vi "Configure.vi"(7 "Task Ident":string, 8 "error in":errorcluster, 9 "Task-Point Idents":string[](array[string]), 10 "MSS":refnum<class "Measure and Stimulus Subsystems.lvclass">, 11 "ITask Actor in":refnum<class "Task Actor.lvclass">) -> (0 "error out":errorcluster, 3 "ITask Actor out":refnum<class "Task Actor.lvclass">)   [LabVIEW 2023, in "Task Actor.lvlib" / "Task Actor.lvclass"]
uses:
  Task Actor.lvclass
  Measure and Stimulus Subsystems/Measure and Stimulus Subsystems.lvclass
  Task Actor.lvclass/Task Actor.ctl
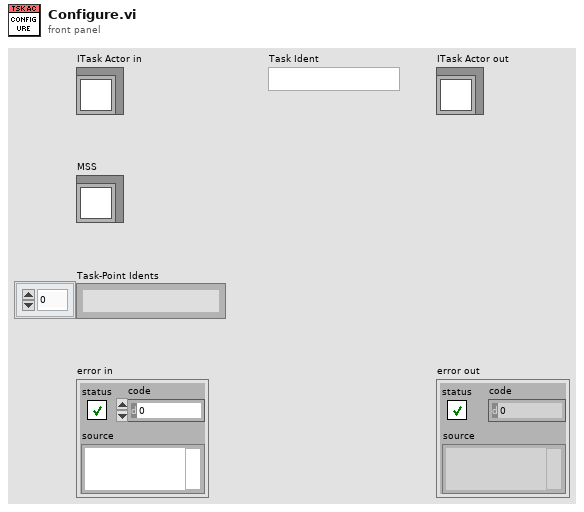
[diagram p1: front panel]
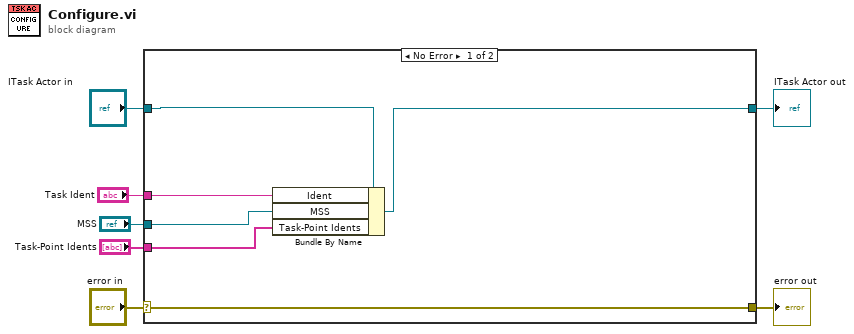
[diagram p0: block diagram]
diagram:
  n1 = case shown="No Error" "error in" {
    selector: "error in" -> [w13 w15]
    tunnel: [w13 w15] -> w6
    tunnel: [w11 w14] -> w4
    tunnel: "ITask Actor in" -> [w12 w14]
    tunnel: "Task Ident" -> [w10 _]
    tunnel: "MSS" -> [w9 _]
    tunnel: "Task-Point Idents" -> [w8 _]
    frame No Error {
      n2 = Bundle By Name(cluster=w12, "Ident"=w10, "MSS"=w9, "Task-Point Idents"=w8) -> (w11:refnum<class "Task Actor.lvclass">)
    }
    frame Error {
    }
  }
  "error out" <- w6
  "ITask Actor out" <- w4
